vi "Choose Correct Instrument.vi"(1 "Instrument Keys":string[](array[string]), 3 "error in (no error)":errorcluster) -> (8 "Selected Instrument Key":string, 10 "error out":errorcluster)   [LabVIEW 2016, in "Drivers.lvlib" / "Agilis.lvlib"]
uses:
  Agilis.lvlib
panel:
  in  "select my instrument":bool
  in  "Instrument Keys List":u16(ring) items=["COM1", "COM4"]
  # "If you have instruments connected but still the list is blank, then \nverify that the command library reference is properly passed\nfrom the constructor node (in Open.vi) to the other wire terminals."
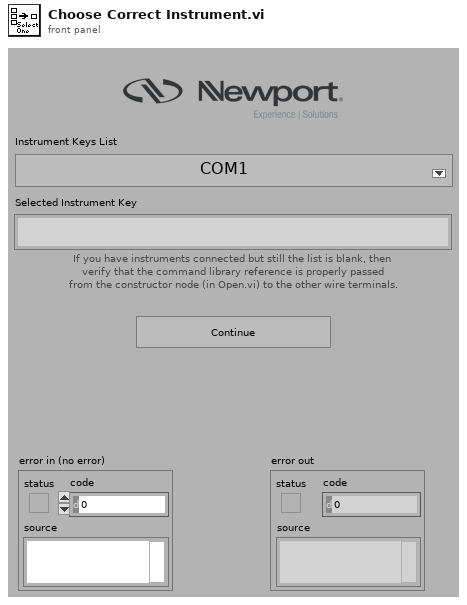
[diagram p1: front panel]
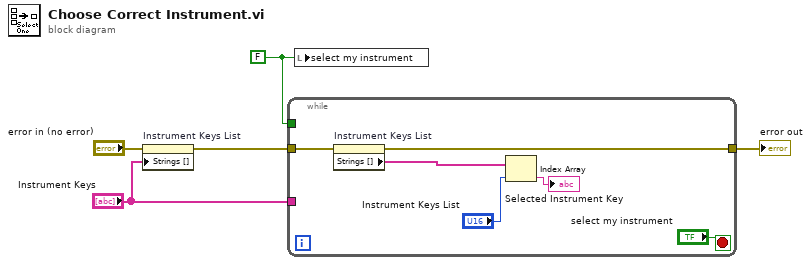
[diagram p0: block diagram]
diagram:
  w4 = FALSE ("stop")
  n1 = property on="Instrument Keys List" class="Ring (strict)"(error in="error in (no error)", "Strings []"="Instrument Keys") -> (error out=w2:errorcluster)  [unwired: 1 in, 1 out]
  n2 = while {
    tunnel: "Instrument Keys" -> [_]
    tunnel: w4 -> [_]
    tunnel: w2 -> [w7]
    tunnel: [w6] -> w1
    stop <- "select my instrument" stop-if-true
    n3 = property on="Instrument Keys List" class="Ring (strict)"(error in=w7) -> (error out=w6:errorcluster, "Strings []"=w10:string[])  [unwired: 1 in, 1 out]
    n4 = Index Array(array=w10, index="Instrument Keys List") -> (element=→"Selected Instrument Key":string)
  }
  "error out" <- w1
  n5 = local write "select my instrument"(w4) -> ()
